vi "Wait For Position.vi"(4 "error in (no error)":errorcluster, 5 "Position (0 units)":dbl format="%.4f", 6 "Axis (1)":i32=1 min=1 max=3, 7 "VISA resource name":refnum<visa-resource-name>) -> (0 "error out":errorcluster, 3 "VISA resource name out":refnum<visa-resource-name>)   [LabVIEW 2019, in "Newport ESP301.lvlib"]
doc: "This command stops program execution until a user specified position is reached. The program continues executing any subsequent commands only after axis Axis (1) has reached position Position (0 units).\nNote:\nEnsure that position Position (0 units) is within the travel range of axis Axis (1). The controller cannot always detect if a value is outside the travel range of an axis to flag an error, especially while making coordinated motion of multiple axes.\nWait commands are primarily intended for use in internal program execution or in combination with the RQ command. If used in command mode, it is important to note that input command processing is suspended until the wait condition has been satisfied."
uses:
  Newport ESP301.lvlib
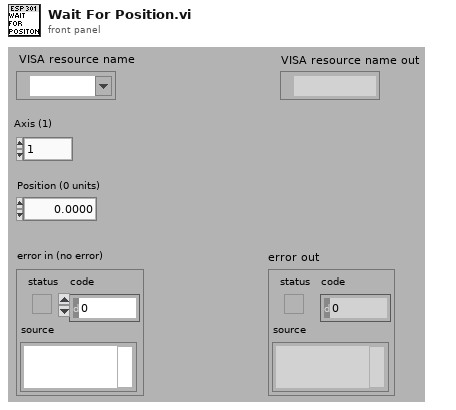
[diagram p1: front panel]
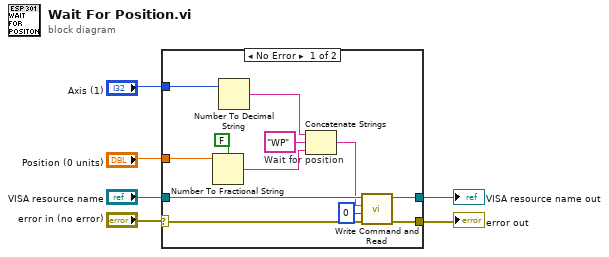
[diagram p0: block diagram]
diagram:
  n1 = case shown="No Error" "error in (no error)" {
    selector: "error in (no error)" -> [w15 w20]
    tunnel: [w17 w20] -> w6
    tunnel: "VISA resource name" -> [w18 w19]
    tunnel: [w16 w19] -> w5
    tunnel: "Axis (1)" -> [w10 _]
    tunnel: "Position (0 units)" -> [w9 _]
    frame No Error {
      w14 = "WP"  # Wait for position
      n2 = Number To Fractional String(use system decimal point (T)=FALSE ("utiliser le séparateur décimal du système (V)"), number=w9) -> (F-format string=w13:string)  [unwired: 2 in]
      n3 = Number To Decimal String(number=w10) -> (decimal integer string=w12:string)  [unwired: 1 in]
      n4 = Concatenate Strings(w12, w14, w13) -> (w11:string)
      n5 = call "Write Command and Read.vi"("error in (no error)"=w15, "Bytes to read (100)"=u32 0, "Command"=w11, "VISA resource name"=w18) -> ("error out"=w17:errorcluster, "VISA resource name out"=w16:refnum<visa-resource-name>)  [unwired: 3 in, 1 out]
    }
    frame Error {
    }
  }
  "error out" <- w6
  "VISA resource name out" <- w5
